vi "HelloWorldTest.vi"() -> (0 "Array of Error Description":T1)   [LabVIEW 2019]
uses:
  TestUtility/utility.llb/array of error description.ctl
  TestUtility/utility.llb/error description.ctl
  TestUtility/utility.llb/error type.ctl
panel:
  out "Pass":bool
  in  "error in (no error)":errorcluster
  in  "Server VI path":path=path "../../examples/helloworld/helloworld_server/Run greeter_server.vi"
  in  "Client VI Path":path=path "../../examples/helloworld/helloworld_client/Run greeter_client.vi"
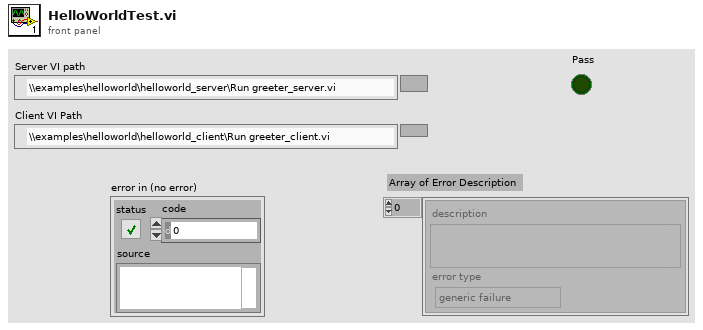
[diagram p1: front panel]
types:
  T1 = typedef "array of error description.ctl" = T2[]
  T2 = typedef "error description.ctl" = cluster{"description":string, "error type":T3}
  T3 = typedef "error type.ctl" = enum32{"generic failure", "boundary case", "precision", "expected error"}
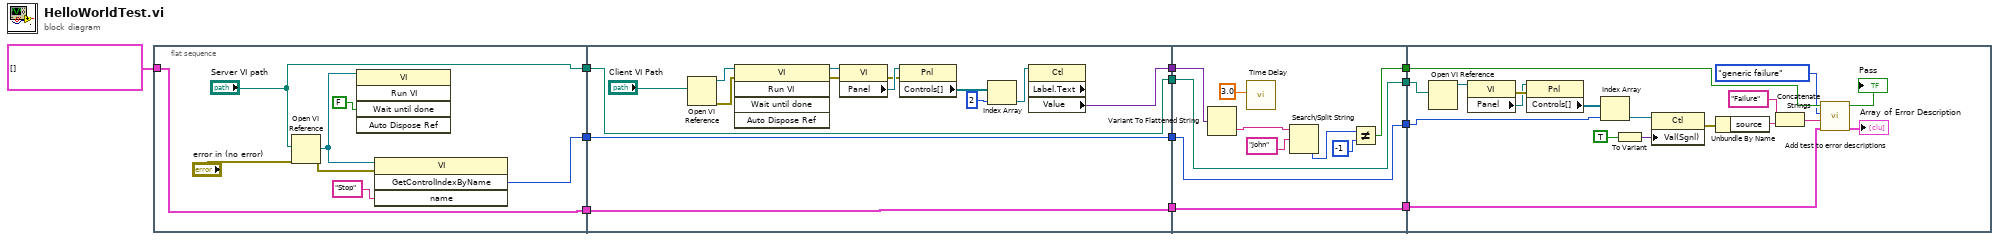
[diagram p0: block diagram]
diagram:
  n1 = flat-sequence {
    tunnel: [w16] -> w11
    tunnel: ["Server VI path"] -> w10
    tunnel: T1 [] ("error descriptions in") -> [w13]
    tunnel: [w13] -> w3
    tunnel: [w34] -> w12
    tunnel: w11 -> [w22]
    tunnel: w10 -> [w23]
    tunnel: [w23] -> w9
    tunnel: [w22] -> w7
    tunnel: w3 -> [w21]
    tunnel: [w21] -> w2
    tunnel: w12 -> [w42]
    tunnel: w9 -> [w40]
    tunnel: [w40] -> w8
    tunnel: w7 -> [w39]
    tunnel: [w39] -> w6
    tunnel: [w37] -> w5
    tunnel: w2 -> [w36]
    tunnel: [w36] -> w1
    tunnel: w8 -> [w61]
    tunnel: w6 -> [w56]
    tunnel: w5 -> [w51]
    tunnel: w1 -> [w45]
    frame #0 {
      n2 = Open VI Reference(vi path="Server VI path", error in (no error)="error in (no error)") -> (vi reference=w15:refnum<vi>, error out=w19:errorcluster)  [unwired: 4 in]
      n3 = invoke class="VI" method="Run VI"(reference=w15, "Wait until done"=FALSE ("Wait Until Done")) -> ()  [unwired: 3 in, 5 out]
      n4 = invoke class="VI" method="GetControlIndexByName"(reference=w15, error in=w19, "name"="Stop" ("Control Name")) -> ("GetControlIndexByName"=w16:i32)  [unwired: 1 in, 3 out]
    }
    frame #1 {
      n5 = Open VI Reference(vi path="Client VI Path") -> (vi reference=w32:refnum<vi>, error out=w31:errorcluster)  [unwired: 5 in]
      n6 = invoke class="VI" method="Run VI"(reference=w32, error in=w31) -> (reference out=w30:refnum<vi>, error out=w29:errorcluster)  [unwired: 3 in, 3 out]
      n7 = property class="VI"(reference=w30, error in=w29) -> (error out=w27:errorcluster, "Panel"=w28:refnum<vi>)  [unwired: 1 out]
      n8 = property class="Pnl"(reference=w28, error in=w27) -> ("Controls[]"=w26:refnum<vi>[])  [unwired: 2 out]
      n9 = Index Array(array=w26, index=2) -> (element=w24:refnum<vi>)
      n10 = property class="Ctl" props=["Label", "Text", "Value"](reference=w24) -> ("Value"=w34:variant)  [unwired: 1 in, 3 out]
    }
    frame #2 {
      n11 = Variant To Flattened String(Variant=w42) -> (data string=w43:string)  [unwired: 1 out]
      n12 = call "Time Delay"("Delay Time (s)"=3.0) -> ()  [unwired: 10 in, 1 out]
      n13 = Search/Split String(string=w43, search string/char (-)="John") -> (offset of match=w38:i32)  [unwired: 1 in, 2 out]
      n14 = Not Equal?(x=w38, y=-1) -> (x != y?=w37:bool)
    }
    frame #3 {
      n15 = Open VI Reference(vi path=w61) -> (vi reference=w60:refnum<vi>)  [unwired: 5 in, 1 out]
      n16 = property class="VI"(reference=w60) -> (error out=w59:errorcluster, "Panel"=w58:refnum<vi>)  [unwired: 1 in, 1 out]
      n17 = property class="Pnl"(reference=w58, error in=w59) -> ("Controls[]"=w57:refnum<vi>[])  [unwired: 2 out]
      n18 = Index Array(array=w57, index=w56) -> (element=w55:refnum<vi>)
      n19 = To Variant(anything=TRUE) -> (Variant=w54:variant)
      n20 = property class="Ctl"(reference=w55, "Val(Sgnl)"=w54) -> (error out=w48:errorcluster)  [unwired: 1 in, 1 out]
      n21 = Unbundle By Name(w48) -> ("source"=w47:string)
      n22 = Concatenate Strings("Failure" ("string"), w47) -> (w49:string)
      n23 = call "Add test to error descriptions.vi"("error descriptions in"=w45, "error string"=w49, "error type"=error_type."generic failure", "pass"=w51) -> ("error description out"=→"Array of Error Description":T1)  [unwired: 3 in]
      "Pass" <- w51
    }
  }
